vi "Evaluate Part 1.vi"() -> ()   [LabVIEW 2020]
uses:
  Galaxy/Galaxy.lvclass
panel:
  out "sum 2":i32
  out "sum":i32
  in  "Input":string
  # "9693756"
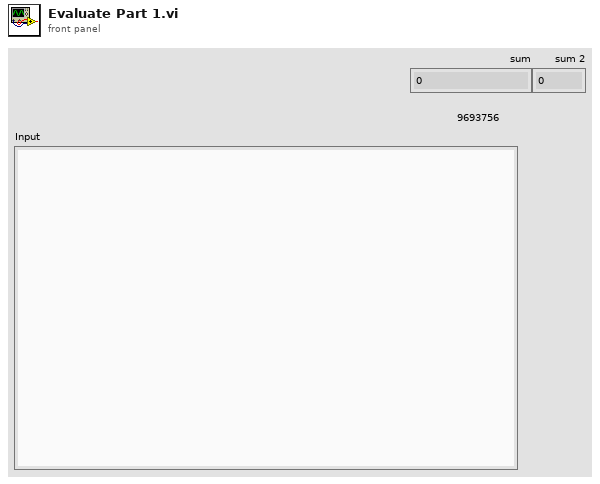
[diagram p1: front panel]
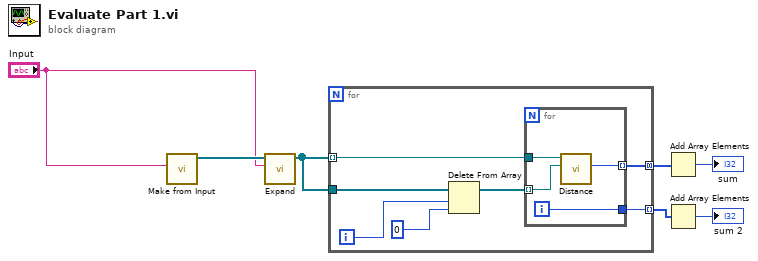
[diagram p0: block diagram]
diagram:
  n1 = call "Make from Input.vi"("Input"="Input") -> ("Galaxy out"=w7:refnum<class "Galaxy.lvclass">[])  [unwired: 9 in, 1 out]
  n2 = call "Expand.vi"("Input"="Input", "Galaxy in"=w7) -> ("Array"=w5:refnum<class "Galaxy.lvclass">[])  [unwired: 8 in, 1 out]
  n3 = for {
    tunnel: w5 -> [w14] mode=indexing
    tunnel: w5 -> [w13]
    tunnel: [w9] -> w4 mode=concatenating
    tunnel: [w8] -> w2 mode=indexing
    i -> [w12]
    n4 = Delete From Array(array=w13, length=w12, index=0) -> (array with subset deleted=w10:refnum<class "Galaxy.lvclass">[])  [unwired: 1 out]
    n5 = for {
      tunnel: w14 -> [w18]
      tunnel: w10 -> [w17] mode=indexing
      tunnel: [w16] -> w9 mode=indexing
      tunnel: [w15] -> w8
      i -> [w15]
      n6 = call "Distance.vi"("Galaxy in 2"=w17, "Galaxy in"=w18) -> ("Numeric"=w16:i64)  [unwired: 8 in, 1 out]
    }
  }
  n7 = Add Array Elements(numeric array=w4) -> (sum=→"sum":i64)
  n8 = Add Array Elements(numeric array=w2) -> (sum=→"sum 2":i32)
